vi "Run.vi"(0 "reference in":refnum<class "ConveyorBelt.lvclass">, 5 "error in (no error)":errorcluster) -> (14 "reference out":refnum<class "ConveyorBelt.lvclass">, 19 "error out":errorcluster)   [LabVIEW 2014, in "ConveyorBelt.lvclass"]
uses:
  ConveyorBelt.lvclass
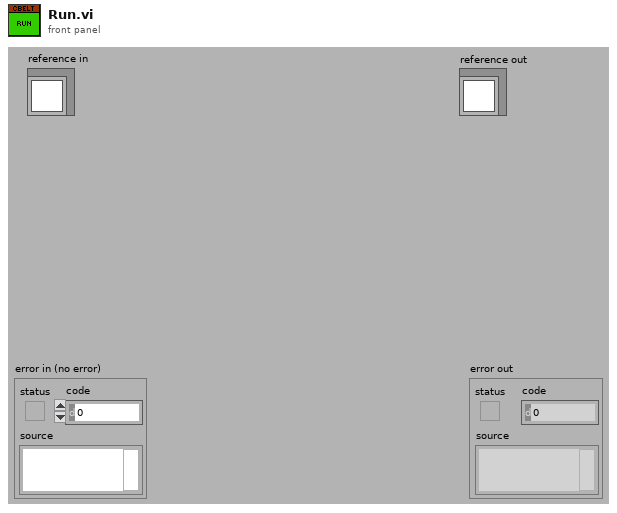
[diagram p1: front panel]
types:
  T1 = typedef "ConveyorBelt.lvclass/ObjectAttributes.ctl" = cluster{"Right":bool, "Running":bool, "ConveyorBeltRef":refnum<vi>}
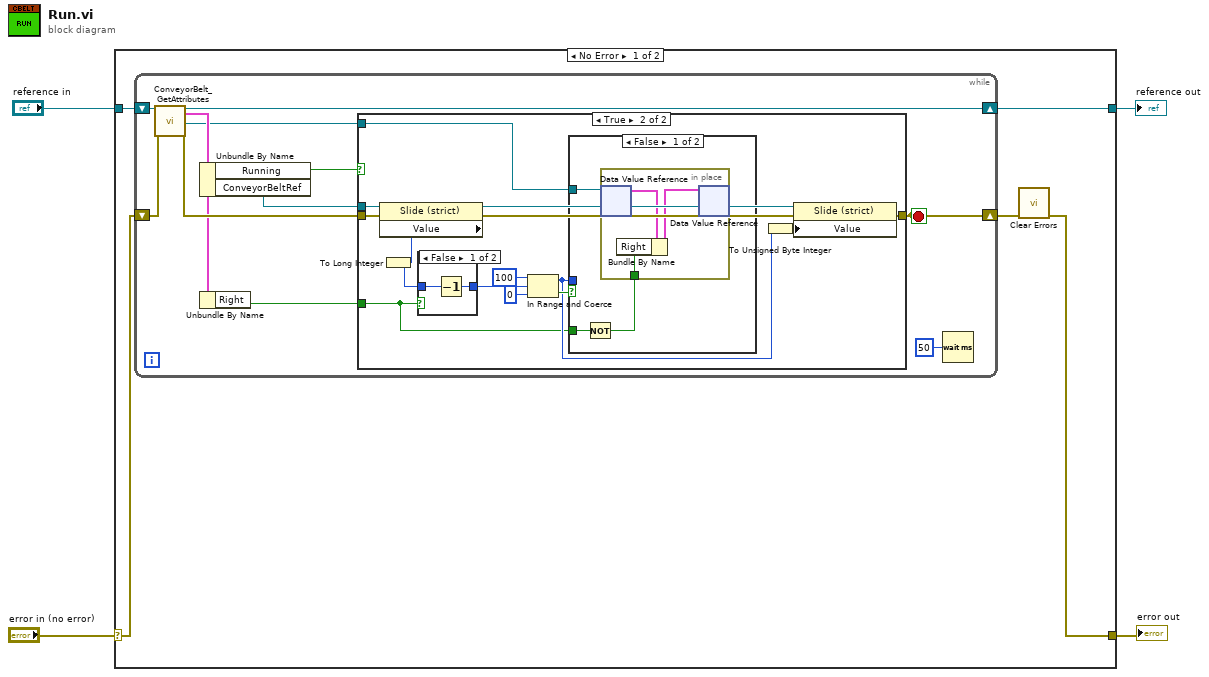
[diagram p0: block diagram]
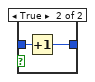
[diagram p3: hidden frame]
diagram:
  n1 = case shown="No Error" "error in (no error)" {
    selector: "error in (no error)" -> [w9 w47]
    tunnel: [w5 w47] -> w3
    tunnel: [w7 w46] -> w1
    tunnel: "reference in" -> [w8 w46]
    frame No Error {
      n2 = while {
        shift-right: [w15] -> w6
        shift-left: w9 -> [w18]
        shift-right: [w19] -> w7
        shift-left: w8 -> [w20]
        stop <- w15 stop-if-true
        n3 = call "ConveyorBelt_GetAttributes.vi"("reference in"=w20, "error in (no error)"=w18) -> ("reference out"=w19:refnum<class "ConveyorBelt.lvclass">, "Data"=w12:T1, "DataRef"=w10:refnum<data-value>, "error out"=w16:errorcluster)  [unwired: 14 in]
        n4 = Unbundle By Name(w12) -> ("Running"=w13:bool, "ConveyorBeltRef"=w14:refnum<vi>)
        n5 = Unbundle By Name(w12) -> ("Right"=w11:bool)
        n6 = case shown="True" w13 {
          tunnel: w16 -> [w21 w35]
          tunnel: [w21 w34] -> w15
          tunnel: w14 -> [_ w33]
          tunnel: w11 -> [_ w24]
          tunnel: w10 -> [_ w25]
          frame False {
          }
          frame True {
            n7 = property class="Slide (strict)"(reference=w33, error in=w35) -> (reference out=w32:refnum<vi>, error out=w34:errorcluster, "Value"=w29:u8)
            n8 = To Long Integer(number=w29) -> (32bit integer=w23:i32)
            n9 = case shown="False" w24 {
              tunnel: w23 -> [w37 w39]
              tunnel: [w36 w38] -> w28
              frame False {
                n10 = Decrement(x=w37) -> (x-1=w36:i32)
              }
              frame True {
                n11 = Increment(x=w39) -> (x+1=w38:i32)
              }
            }
            n12 = In Range and Coerce(upper limit=100, x=w28, lower limit=0) -> (coerced(x)=w26:i32, In Range?=w27:bool)
            n13 = case shown="False" w27 {
              tunnel: w26 -> [_ _]
              tunnel: w25 -> [w42 _]
              tunnel: w24 -> [w41 _]
              frame False {
                n14 = Not(x=w41) -> (.not. x?=w40:bool)
                n15 = in-place {
                  in-place-border: w40 -> [w43]
                  n16 = in-place-dvr #1(w42) -> (w45:T1)  [unwired: 1 out]
                  n17 = Bundle By Name(cluster=w45, "Right"=w43) -> (w44:T1)
                  n18 = in-place-dvr #1(w44) -> ()  [unwired: 2 out]
                }
              }
              frame True {
              }
            }
            n19 = To Unsigned Byte Integer(number=w26) -> (unsigned 8bit integer=w22:u8)
            n20 = property class="Slide (strict)"(reference=w32, error in=w34, "Value"=w22) -> ()  [unwired: 2 out]
          }
        }
        n21 = Wait (ms)(milliseconds to wait=u32 50) -> ()  [unwired: 1 out]
      }
      n22 = call <vilib>:"Clear Errors.vi"("error in (no error)"=w6) -> ("error out"=w5:errorcluster)  [unwired: 5 in, 1 out]
    }
    frame Error {
    }
  }
  "error out" <- w3
  "reference out" <- w1
